vi "FPGA_Main.vi"() -> ()   [LabVIEW 2013]
uses:
  <vilib>/rvi/Emulation/niFpgaSctlEmulationGetInTimedLoop.vi
  <vilib>/rvi/Emulation/niFpgaEmulationReportErrorSimple.vi
  <vilib>/rvi/Emulation/niFpgaGetClockAttributes.vi
  <vilib>/rvi/Memory/Memory_Emulation/nirvimemoryFastEmulationFpgaImpl.vi
  <instcachedir>/0/nirvimemoryFastEmulationFpgaImpl_5FBAB50466BC4C939F684F8805638BFC.lvgen/nirvimemoryFastEmulationFpgaImpl_5FBAB50466BC4C939F684F8805638BFC_003.vi
  <vilib>/rvi/DataTransferAndStorage/Container/Common/niFpgaContainerGetUniqueNameForEmu.vi
  <vilib>/rvi/Memory/Memory_Emulation/nirvimemoryFastEmulation.vi
  <vilib>/rvi/Memory/Memory_Emulation/nirvimemoryEmulation.vi
  <instcachedir>/0/nirvimemoryFastEmulationFpgaImpl_5FBAB50466BC4C939F684F8805638BFC.lvgen/nirvimemoryFastEmulationFpgaImpl_5FBAB50466BC4C939F684F8805638BFC_005.vi
  <vilib>/rvi/FIFO/Fifo_Resource/nirvififoEmulationReadFpgaImpl.vi
  <vilib>/rvi/eio/common/nirviEmuTemplateMethod_errors.vi
  <vilib>/rvi/interface/RandomDataEmulation/nirviRandomDataFPGAFIFO.vi
  <vilib>/rvi/interface/RandomDataEmulation/niFpgaRandomDataHandleErrors.vi
  <vilib>/rvi/Emulation/niFpgaCriticalErrorInLSC.vi
  <vilib>/rvi/DataTransferAndStorage/Container/XNode/niFpgaContainer.xnode
  <vilib>/rvi/FIFO/Fifo_Resource/nirvififoEmulationRead.vi
  <vilib>/eio/EIONode/EIONode.xnode
  <vilib>/rvi/interface/RandomDataEmulation/nirviRandomDataFpgaReadWriteTemplate.vi
panel:
  in  "tag_ActuationMode":i32
  in  "tag_ClampMode":i32
  out "Derivative":fxp<+/-,50,35>
  out "RunningSum":fxp<+/-,32,8>
  out "Error":fxp<+/-,21,6>
  out "Actuating":bool
  out "Loop Timing (us)":u32
  in  "AntiWindupInterval":fxp<+,20,4>=5.0
  in  "Dgain":fxp<+,32,8>
  in  "Igain":fxp<+,24,12>
  in  "Pgain":fxp<+,24,8>
  in  "tag_ManualSetPoint":fxp<+/-,20,5>
  in  "tag_ActuationFreq":i32=100
  in  "tag_AcqFreq":i32=100
  out "FIFO Full":bool
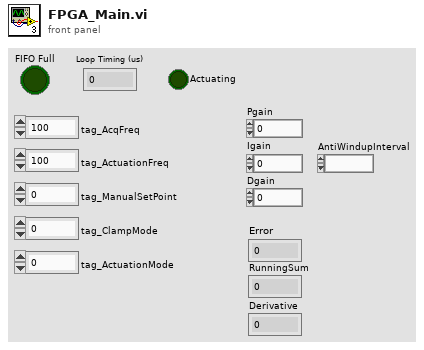
[diagram p1: front panel]
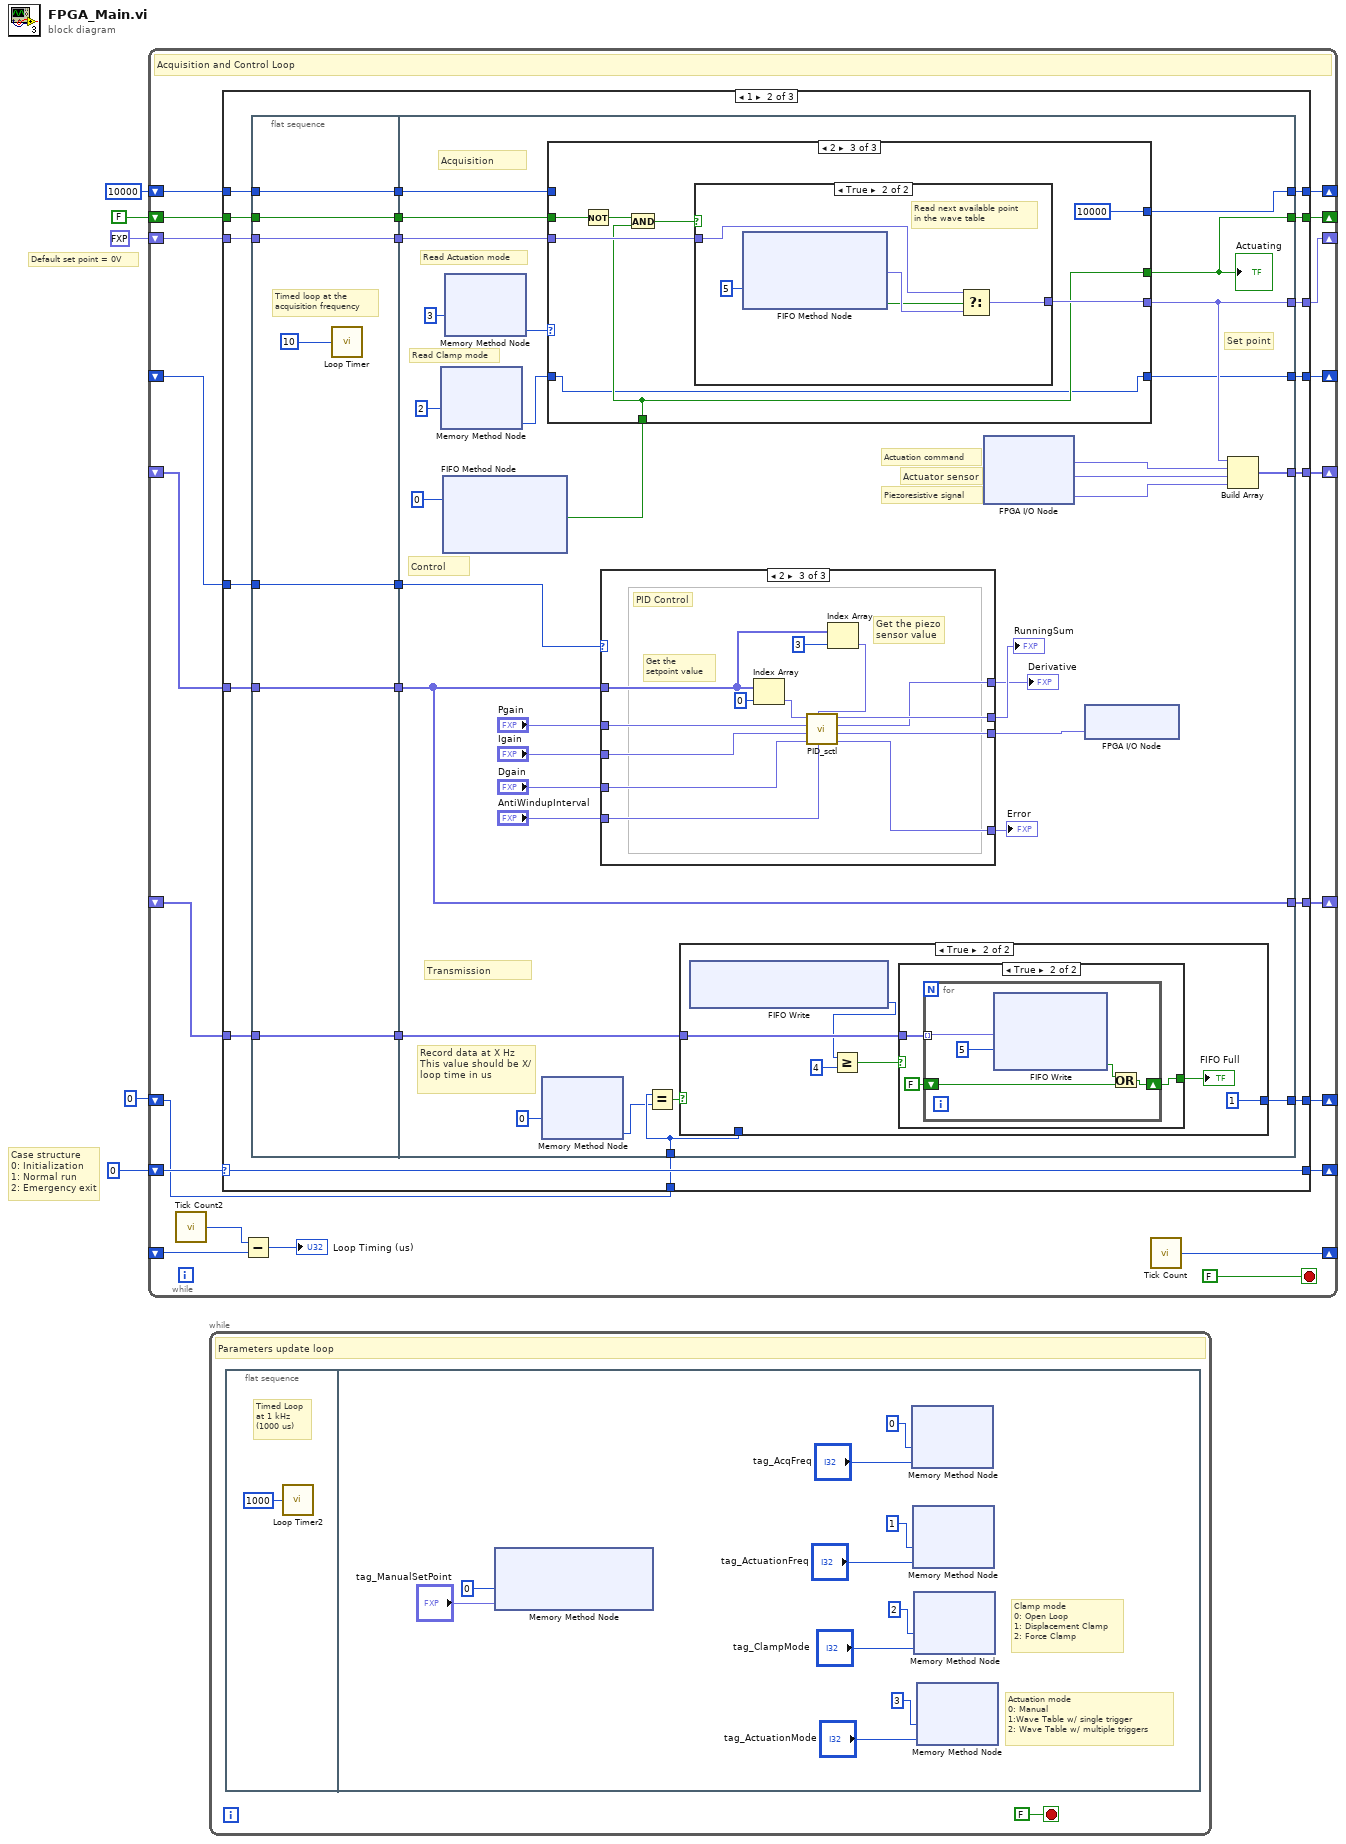
[diagram p0: block diagram]
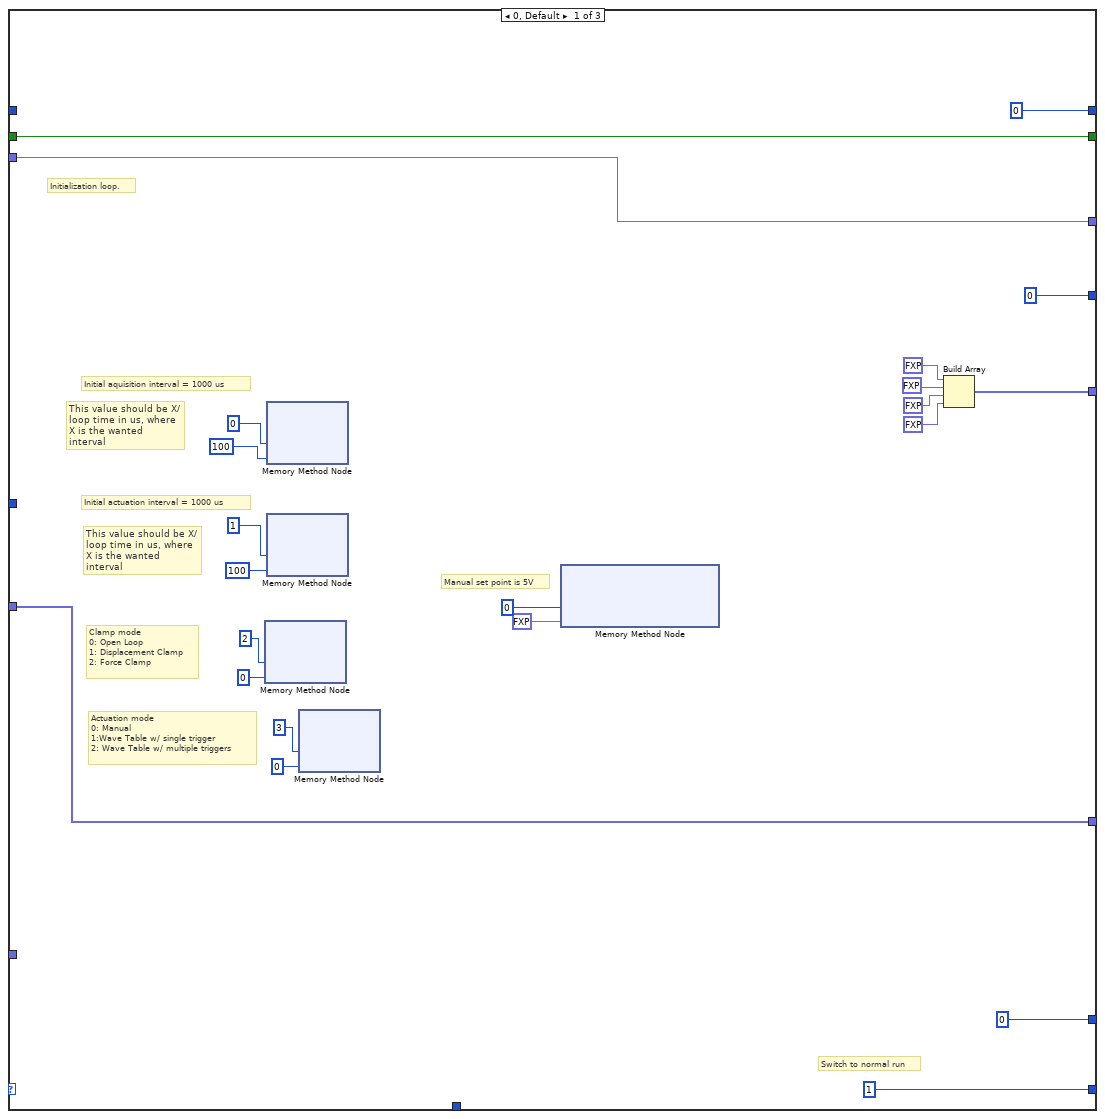
[diagram p2: hidden frame]
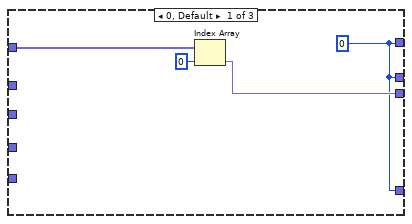
[diagram p3: hidden frame]
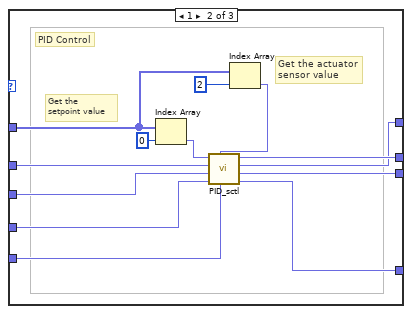
[diagram p4: hidden frame]
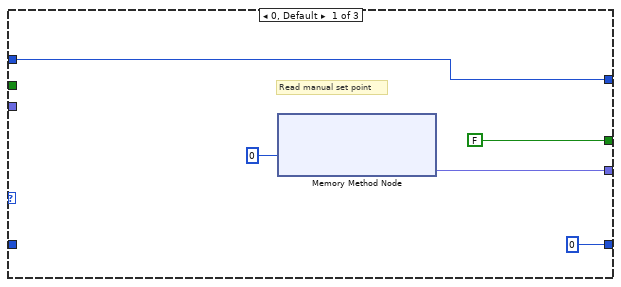
[diagram p5: hidden frame]
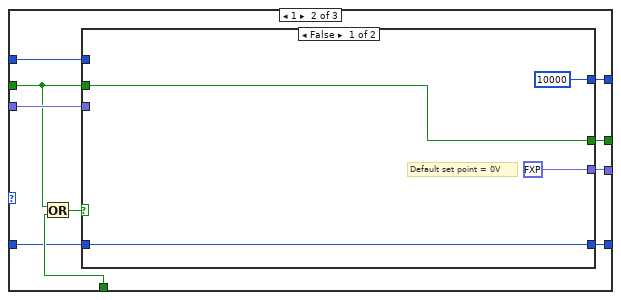
[diagram p6: hidden frame]
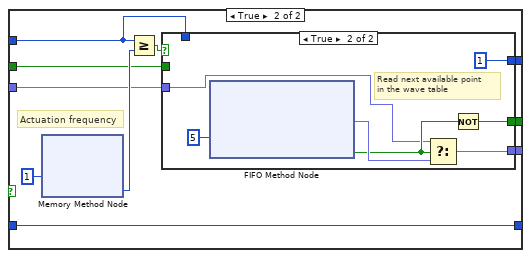
[diagram p7: hidden frame]
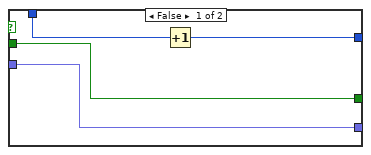
[diagram p8: hidden frame]
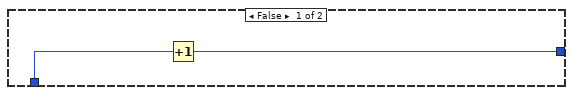
[diagram p10: hidden frame]
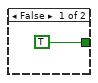
[diagram p11: hidden frame]
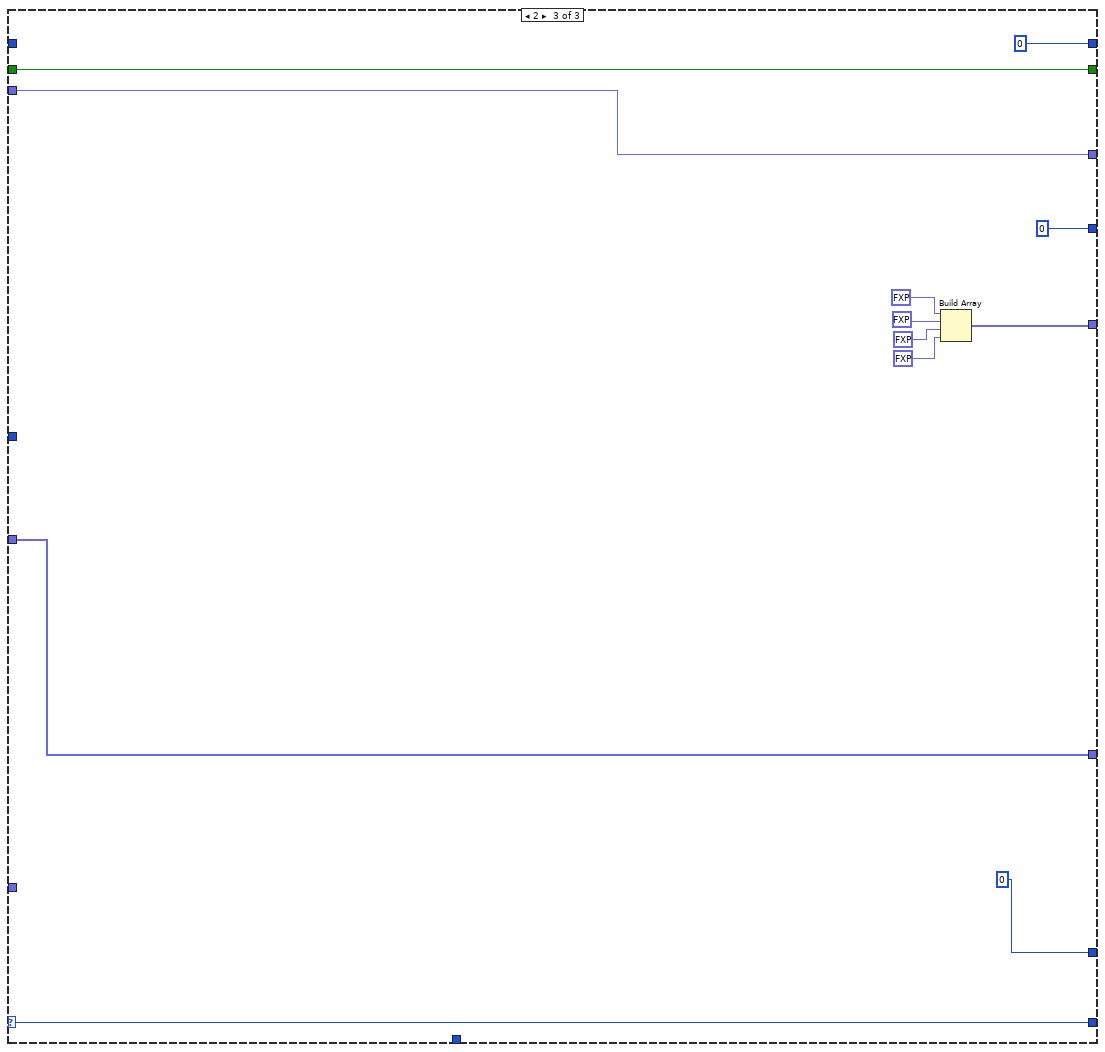
[diagram p12: hidden frame]
diagram:
  # "Default set point = 0V"
  # "Case structure\n0: Initialization\n1: Normal run\n2: Emergency exit"
  n1 = while {
    shift-right: [w24] -> _
    shift-left: i16 0 -> [w25]
    shift-right: [w23] -> _
    shift-left: _ -> [w20]
    shift-right: [w22] -> _
    shift-left: _ -> [w21]
    shift-right: [w19] -> _
    shift-left: _ -> [w17]
    shift-right: [w15] -> _
    shift-left: FALSE -> [w14]
    shift-right: [w8] -> _
    shift-left: fxp<+/-,20,5> 0.0 -> [w13]
    shift-right: [w11] -> _
    shift-left: u16 0 -> [w12]
    shift-right: [w10] -> _
    shift-left: u16 10000 -> [w9]
    shift-right: [w7] -> _
    shift-left: _ -> [w6]
    stop <- FALSE stop-if-true
    # "Acquisition and Control Loop"
    n2 = call "Tick Count2"() -> ("Tick Count(uSec)"=w18:u32)
    n3 = case shown="1" w25 {
      selector: w25 -> [_ w69 w222]
      tunnel: [i16 1 w69 w222] -> w24
      tunnel: [w39 w68 w217] -> w23
      tunnel: [w43 w67 w221] -> w22
      tunnel: w20 -> [w43 w65 w221]
      tunnel: w21 -> [_ w63 _]
      tunnel: [w37 w62 w215] -> w15
      tunnel: w14 -> [w37 w60 w215]
      tunnel: [w36 w59 w214] -> w8
      tunnel: w13 -> [w36 w57 w214]
      tunnel: w12 -> [_ w56 _]
      tunnel: [u8 0 w55 u8 0] -> w11
      tunnel: [u16 0 w54 u16 0] -> w10
      tunnel: w9 -> [_ w52 _]
      tunnel: [u16 0 w51 u16 0] -> w7
      tunnel: w6 -> [_ w49 _]
      frame 0, Default {
        # "Actuation mode\n0: Manual\n1:Wave Table w/ single trigger\n2: Wave Table w/ multiple triggers"
        # "This value should be X/loop time in us, where X is the wanted interval"
        # "This value should be X/loop time in us, where X is the wanted interval"
        # "Clamp mode\n0: Open Loop\n1: Displacement Clamp\n2: Force Clamp"
        # "Manual set point is 5V"
        # "Switch to normal run"
        # "Initial actuation interval = 1000 us"
        # "Initial aquisition interval = 1000 us"
        # "Initialization loop."
        n4 = xnode ("Memory Method Node")("Address"=i16 2, "Data"=i16 0) -> ()  [unwired: 1 in, 1 out]
        n5 = xnode ("Memory Method Node")("Address"=i16 0, "Data"=i16 100) -> ()  [unwired: 1 in, 1 out]
        n6 = xnode ("Memory Method Node")("Address"=i16 1, "Data"=i16 100) -> ()  [unwired: 1 in, 1 out]
        n7 = xnode ("Memory Method Node")("Address"=i16 3, "Data"=i16 0) -> ()  [unwired: 1 in, 1 out]
        n8 = xnode ("Memory Method Node")("Address"=i16 0, "Data"=fxp<+/-,20,5> 5.0) -> ()  [unwired: 1 in, 1 out]
        n9 = Build Array(fxp<+/-,20,5> 0.0, fxp<+/-,20,5> 0.0, fxp<+/-,20,5> 0.0, fxp<+/-,20,5> 0.0) -> (w39:fxp<+/-,20,5>[])
      }
      frame 1 {
        n10 = flat-sequence {
          tunnel: [w76] -> w66
          tunnel: w65 -> [w76]
          tunnel: [w75] -> w64
          tunnel: w63 -> [w75]
          tunnel: [w74] -> w61
          tunnel: w60 -> [w74]
          tunnel: [w73] -> w58
          tunnel: w57 -> [w73]
          tunnel: [w71] -> w53
          tunnel: w52 -> [w71]
          tunnel: [w70] -> w50
          tunnel: w49 -> [w70]
          tunnel: [w98] -> w68
          tunnel: [w107] -> w67
          tunnel: w66 -> [w107]
          tunnel: w64 -> [w109]
          tunnel: [w102] -> w62
          tunnel: w61 -> [w94]
          tunnel: [w97] -> w59
          tunnel: w58 -> [w93]
          tunnel: w56 -> [w106]
          tunnel: [w105] -> w55
          tunnel: [w95] -> w54
          tunnel: w53 -> [w96]
          tunnel: [w79] -> w51
          tunnel: w50 -> [w77]
          frame #0 {
            # "Timed loop at the \nacquisition frequency"
            n11 = call "Loop Timer"("Count(uSec)"=i16 10) -> ()  [unwired: 1 out]
          }
          frame #1 {
            # "Read Clamp mode"
            # "Acquisition"
            # "Set point"
            # "Actuation command"
            # "Piezoresistive signal"
            # "Actuator sensor"
            # "Read Actuation mode"
            # "Transmission"
            # "Control"
            # "Record data at X Hz\nThis value should be X/loop time in us"
            n12 = xnode ("Memory Method Node")("Address"=i16 2) -> ("Data"=w80:i16)  [unwired: 1 in, 1 out]
            n13 = xnode ("FIFO Method Node")("Timeout"=i16 0) -> ("Element"=w78:bool)  [unwired: 1 in, 2 out]
            n14 = xnode ("Memory Method Node")("Address"=i16 3) -> ("Data"=w103:i16)  [unwired: 1 in, 1 out]
            n15 = xnode ("Memory Method Node")("Address"=i16 0) -> ("Data"=w82:i16)  [unwired: 1 in, 1 out]
            n16 = case shown="2" w103 {
              tunnel: [w143 w152 w186] -> w97
              tunnel: [FALSE w153 w181] -> w102
              tunnel: w96 -> [w141 w154 _]
              tunnel: [w141 w151 u16 10000] -> w95
              tunnel: w94 -> [_ w148 w185]
              tunnel: w93 -> [_ w150 w182]
              tunnel: w78 -> [_ w147 w181]
              tunnel: w80 -> [_ w146 w180]
              tunnel: [u16 0 w145 w180] -> w79
              frame 0, Default {
                # "Read manual set point"
                n17 = xnode ("Memory Method Node")("Address"=i16 0) -> ("Data"=w143:fxp<+/-,20,5>)  [unwired: 1 in, 1 out]
              }
              frame 1 {
                n18 = Or(x=w148, y=w147) -> (x .or. y?=w149:bool)
                n19 = case shown="False" w149 {
                  tunnel: w154 -> [_ w163]
                  tunnel: [w157 w165] -> w153
                  tunnel: [fxp<+/-,20,5> 0.0 w164] -> w152
                  tunnel: [u16 10000 w162] -> w151
                  tunnel: w148 -> [w157 w161]
                  tunnel: w150 -> [_ w160]
                  tunnel: [w155 w159] -> w145
                  tunnel: w146 -> [w155 w159]
                  frame False {
                    # "Default set point = 0V"
                  }
                  frame True {
                    # "Actuation frequency"
                    n20 = xnode ("Memory Method Node")("Address"=i16 1) -> ("Data"=w168:i16)  [unwired: 1 in, 1 out]
                    n21 = Greater Or Equal?(x=w163, y=w168) -> (x >= y?=w166:bool)
                    n22 = case shown="True" w166 {
                      tunnel: [w170 w176] -> w165
                      tunnel: [w169 w175] -> w164
                      tunnel: w163 -> [w172 _]
                      tunnel: [w171 i16 1] -> w162
                      tunnel: w161 -> [w170 _]
                      tunnel: w160 -> [w169 w173]
                      frame False {
                        n23 = Increment(x=w172) -> (x+1=w171:u16)
                      }
                      frame True {
                        # "Read next available point\nin the wave table"
                        n24 = xnode ("FIFO Method Node")("Timeout"=i16 5) -> ("Element"=w178:fxp<+/-,20,5>, "Timed Out?"=w177:bool)  [unwired: 1 in, 1 out]
                        n25 = Select(t=w173, s=w177, f=w178) -> (s? t:f=w175:fxp<+/-,20,5>)
                        n26 = Not(x=w177) -> (.not. x?=w176:bool)
                      }
                    }
                  }
                }
              }
              frame 2 {
                n27 = Not(x=w185) -> (.not. x?=w184:bool)
                n28 = And(x=w184, y=w181) -> (x .and. y?=w183:bool)
                n29 = case shown="True" w183 {
                  tunnel: [w188 w190] -> w186
                  tunnel: w182 -> [w188 w189]
                  frame False {
                  }
                  frame True {
                    # "Read next available point\nin the wave table"
                    n30 = xnode ("FIFO Method Node")("Timeout"=i16 5) -> ("Element"=w192:fxp<+/-,20,5>, "Timed Out?"=w191:bool)  [unwired: 1 in, 1 out]
                    n31 = Select(t=w189, s=w191, f=w192) -> (s? t:f=w190:fxp<+/-,20,5>)
                  }
                }
              }
            }
            "Actuating" <- w102
            n32 = case shown="2" w77 {
              tunnel: w107 -> [w112 w122 w135]
              tunnel: [w111 w121 w132] -> w91
              tunnel: "Pgain" -> [_ w120 w127]
              tunnel: "Igain" -> [_ w119 w128]
              tunnel: "Dgain" -> [_ w118 w129]
              tunnel: "AntiWindupInterval" -> [_ w117 w130]
              tunnel: [w110 w116 w134] -> w86
              tunnel: [w110 w115 w133] -> w85
              tunnel: [w110 w114 w131] -> w84
              frame 0, Default {
                w110 = i16 0
                n33 = Index Array(array=w112, index=0) -> (element=w111:fxp<+/-,20,5>)
              }
              frame 1 {
                # "PID Control"
                # "Get the\nsetpoint value"
                # "Get the actuator \nsensor value"
                n34 = Index Array(array=w122, index=i16 0) -> (element=w124:fxp<+/-,20,5>)
                n35 = Index Array(array=w122, index=i16 2) -> (element=w123:fxp<+/-,20,5>)
                n36 = call "PID_sctl.vi"("AntiWindupInterval"=w117, "MeasuredValue"=w123, "Dgain"=w118, "Igain"=w119, "Pgain"=w120, "SetPoint"=w124) -> ("Error"=w114:fxp<+/-,21,6>, "ControlEffort"=w121:fxp<+/-,22,7>, "Derivative"=w115:fxp<+/-,50,35>, "RunningSum"=w116:fxp<+/-,32,8>)  [unwired: 2 in]
              }
              frame 2 {
                # "PID Control"
                # "Get the\nsetpoint value"
                # "Get the piezo \nsensor value"
                n37 = Index Array(array=w135, index=i16 0) -> (element=w137:fxp<+/-,20,5>)
                n38 = Index Array(array=w135, index=i16 3) -> (element=w136:fxp<+/-,20,5>)
                n39 = call "PID_sctl.vi"("AntiWindupInterval"=w130, "MeasuredValue"=w136, "Dgain"=w129, "Igain"=w128, "Pgain"=w127, "SetPoint"=w137) -> ("Error"=w131:fxp<+/-,21,6>, "ControlEffort"=w132:fxp<+/-,22,7>, "Derivative"=w133:fxp<+/-,50,35>, "RunningSum"=w134:fxp<+/-,32,8>)  [unwired: 2 in]
              }
            }
            "RunningSum" <- w86
            "Derivative" <- w85
            "Error" <- w84
            n40 = Equal?(x=w106, y=w82) -> (x = y?=w108:bool)
            n41 = case shown="True" w108 {
              tunnel: w109 -> [_ w201]
              tunnel: w106 -> [w195 _]
              tunnel: [w194 u16 1] -> w105
              frame False {
                n42 = Increment(x=w195) -> (x+1=w194:u16)
              }
              frame True {
                n43 = xnode ("FIFO Write")() -> ("Number of Elements to Write"=w198:u32)  [unwired: 1 in, 1 out]
                n44 = Greater Or Equal?(x=w198, y=u32 4) -> (x >= y?=w199:bool)
                n45 = case shown="True" w199 {
                  tunnel: w201 -> [_ w205]
                  tunnel: [TRUE w203] -> w196
                  frame False {
                  }
                  frame True {
                    n46 = for {
                      tunnel: w205 -> [w210] mode=indexing
                      shift-right: [w207] -> w203
                      shift-left: FALSE -> [w206]
                      n47 = xnode ("FIFO Write")("Element"=w210, "Timeout"=i16 5) -> ("Timed Out?"=w208:bool)  [unwired: 1 in, 1 out]
                      n48 = Or(x=w208, y=w206) -> (x .or. y?=w207:bool)
                    }
                  }
                }
                "FIFO Full" <- w196
              }
            }
            n49 = xnode "FPGA I/O Node"() -> ("Mod2/AI0"=w101:fxp<+/-,20,5>, "Mod2/AI1"=w100:fxp<+/-,20,5>, "Mod2/AI2"=w99:fxp<+/-,20,5>)  [unwired: 3 in, 3 out]
            n50 = xnode "FPGA I/O Node"("Mod1/AO0"=w91) -> ()  [unwired: 1 in, 1 out]
            n51 = Build Array(w97, w101, w100, w99) -> (w98:fxp<+/-,20,5>[])
          }
        }
      }
      frame 2 {
        n52 = Build Array(fxp<+/-,20,5> 0.0, fxp<+/-,20,5> 0.0, fxp<+/-,20,5> 0.0, fxp<+/-,20,5> 0.0) -> (w217:fxp<+/-,20,5>[])
      }
    }
    n53 = Subtract(x=w18, y=w17) -> (x-y=→"Loop Timing (us)":u32)
    n54 = call "Tick Count"() -> ("Tick Count(uSec)"=w19:u32)
  }
  n55 = while {
    stop <- FALSE stop-if-true
    # "Parameters update loop"
    n56 = flat-sequence {
      frame #0 {
        # "Timed Loop\nat 1 kHz\n(1000 us)"
        n57 = call "Loop Timer2"("Count(uSec)"=i16 1000) -> ()  [unwired: 1 out]
      }
      frame #1 {
        # "Actuation mode\n0: Manual\n1:Wave Table w/ single trigger\n2: Wave Table w/ multiple triggers"
        # "Clamp mode\n0: Open Loop\n1: Displacement Clamp\n2: Force Clamp"
        n58 = xnode ("Memory Method Node")("Address"=i16 0, "Data"="tag_ManualSetPoint") -> ()  [unwired: 1 in, 1 out]
        n59 = xnode ("Memory Method Node")("Address"=i16 0, "Data"="tag_AcqFreq") -> ()  [unwired: 1 in, 1 out]
        n60 = xnode ("Memory Method Node")("Address"=i16 1, "Data"="tag_ActuationFreq") -> ()  [unwired: 1 in, 1 out]
        n61 = xnode ("Memory Method Node")("Address"=i16 2, "Data"="tag_ClampMode") -> ()  [unwired: 1 in, 1 out]
        n62 = xnode ("Memory Method Node")("Address"=i16 3, "Data"="tag_ActuationMode") -> ()  [unwired: 1 in, 1 out]
      }
    }
  }
